vi "sub_FEA_Make_M_and K_Matrices_LEMP.vi"(0 "Setup Parameters":T2) -> (14 "Eigenvalues":cdb[](array[numeric]), 15 "Eigenvectors":T1, 16 "M Matrix":dbl[][](array[numeric]), 17 "K Matrix":dbl[][](array[numeric]), 18 "Element Length":dbl)   [LabVIEW 2019]
uses:
  <vilib>/Analysis/Matrix/Datatypes/RealMatrix.ctl
  <vilib>/Analysis/Matrix/NI_Matrix.lvlib
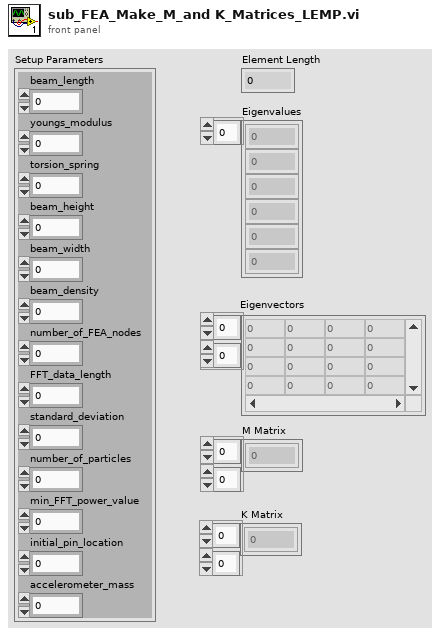
[diagram p1: front panel]
types:
  T1 = typedef "NI_Matrix.lvlib/RealMatrix.ctl" = dbl[][]
  T2 = cluster{"beam_length":dbl, "youngs_modulus":dbl, "torsion_spring":dbl, "beam_height":dbl, "beam_width":dbl, "beam_density":dbl, "number_of_FEA_nodes":i32, "FFT_data_length":i32, "standard_deviation":dbl, "number_of_particles":i32, "min_FFT_power_value":dbl, "initial_pin_location":i32, "accelerometer_mass":dbl}
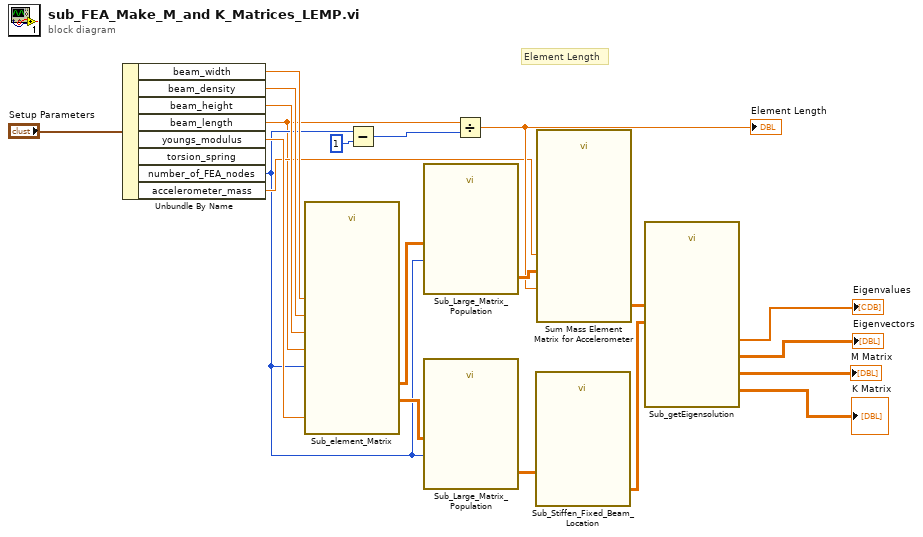
[diagram p0: block diagram]
diagram:
  # "Element Length"
  n1 = Unbundle By Name("Setup Parameters") -> ("beam_width"=w16:dbl, "beam_density"=w17:dbl, "beam_height"=w18:dbl, "beam_length"=w8:dbl, "youngs_modulus"=w19:dbl, "number_of_FEA_nodes"=w9:i32, "accelerometer_mass"=w10:dbl)  [unwired: 1 out]
  n2 = call "Sub_element_Matrix.vi"("Length of Beam"=w8, "Young's Modulus"=w19, "No. of Nodes"=w9, "Height"=w18, "Width"=w16, "Density"=w17) -> ("M Element Matrix"=w20:dbl[][], "K Element Matrix"=w21:dbl[][])  [unwired: 12 in]
  n3 = Subtract(x=w9, y=1) -> (x-y=w14:i32)
  n4 = call "Sub_Large_Matrix_Population.vi"("No. of Nodes"=w9, "Element Matrix"=w20) -> ("Matrix w/o BC"=w15:dbl[][])  [unwired: 9 in]
  n5 = call "Sub_Large_Matrix_Population.vi"("No. of Nodes"=w9, "Element Matrix"=w21) -> ("Matrix w/o BC"=w7:dbl[][])  [unwired: 9 in]
  n6 = Divide(x=w8, y=w14) -> (x/y=w12:dbl)
  "Element Length" <- w12
  n7 = call "Sub_Stiffen_Fixed_Beam_Location.vi"("Pre-BC Matrix"=w7) -> ("Post-BC Matrix"=w5:dbl[][])  [unwired: 10 in]
  n8 = call "Sum Mass Element Matrix for Accelerometer.vi"("Matrix w/o BC"=w15, "accelerometer_mass"=w10, "Element Length"=w12) -> ("Matrix W/ Accelerometer"=w6:dbl[][])  [unwired: 8 in]
  n9 = call "Sub_getEigensolution.vi"("MASS"=w6, "STIFF"=w5) -> ("MASS"=→"M Matrix":T1, "STIFF"=→"K Matrix":T1, "Eigenvectors"=→"Eigenvectors":T1, "Eigenvalues"=→"Eigenvalues":cdb[])  [unwired: 6 in]
